vi "cm2nm_index_fiducials.vi"(2 "CurrentSessionCollectionOfPoints":T1[](array[typedef]), 4 "ReferenceSessionCollectionOfPoints":T1[](array[typedef]), 5 "IndexCurrentSession_PairingList":i32[](array[numeric]), 6 "ReplacePairedFidName":bool, 9 "IndexRefrenceSession_PairlingList":i32[](array[numeric])) -> (0 "CurrentSessionOut":T1[](array[typedef])=[{"MetaDataFile"=path "", "X"=-1.1, "Y"=0.0, "Z"=0.0, "Group"=0, "Rotation"=0.0, "Fiducial"=TRUE, "Magnification"=0.0, "Working_Distance"=0.0, "Notes"="", "Location Name/ID"="", "OtherRelatedDataFiles"=[], "Available"=FALSE}, {"MetaDataFile"=path "", "X"=0.0, "Y"=-1.0, "Z"=0.0, "Group"=0, "Rotation"=0.0, "Fiducial"=TRUE, "Magnification"=0.0, "Working_Distance"=0.0, "Notes"="", "Location Name/ID"="", "OtherRelatedDataFiles"=[], "Available"=FALSE}, {"MetaDataFile"=path "", "X"=0.0, "Y"=1.0, "Z"=0.0, "Group"=0, "Rotation"=0.0, "Fiducial"=TRUE, "Magnification"=0.0, "Working_Distance"=0.0, "Notes"="", "Location Name/ID"="", "OtherRelatedDataFiles"=[], "Available"=FALSE}, {"MetaDataFile"=path "", "X"=1.0, "Y"=0.0, "Z"=0.0, "Group"=0, "Rotation"=0.0, "Fiducial"=TRUE, "Magnification"=0.0, "Working_Distance"=0.0, "Notes"="", "Location Name/ID"="", "OtherRelatedDataFiles"=[], "Available"=FALSE}], 1 "PairedFiducialNames":T2(array[cluster]), 3 "PairedFiducials":T3(array[cluster]))   [LabVIEW 2011]
doc: "This Vi extracts the paired coordinates and names and puts into the format that the coordinate transform functions where created. Just book keeping."
uses:
  cm2nm_coordinate_information_v2.ctl
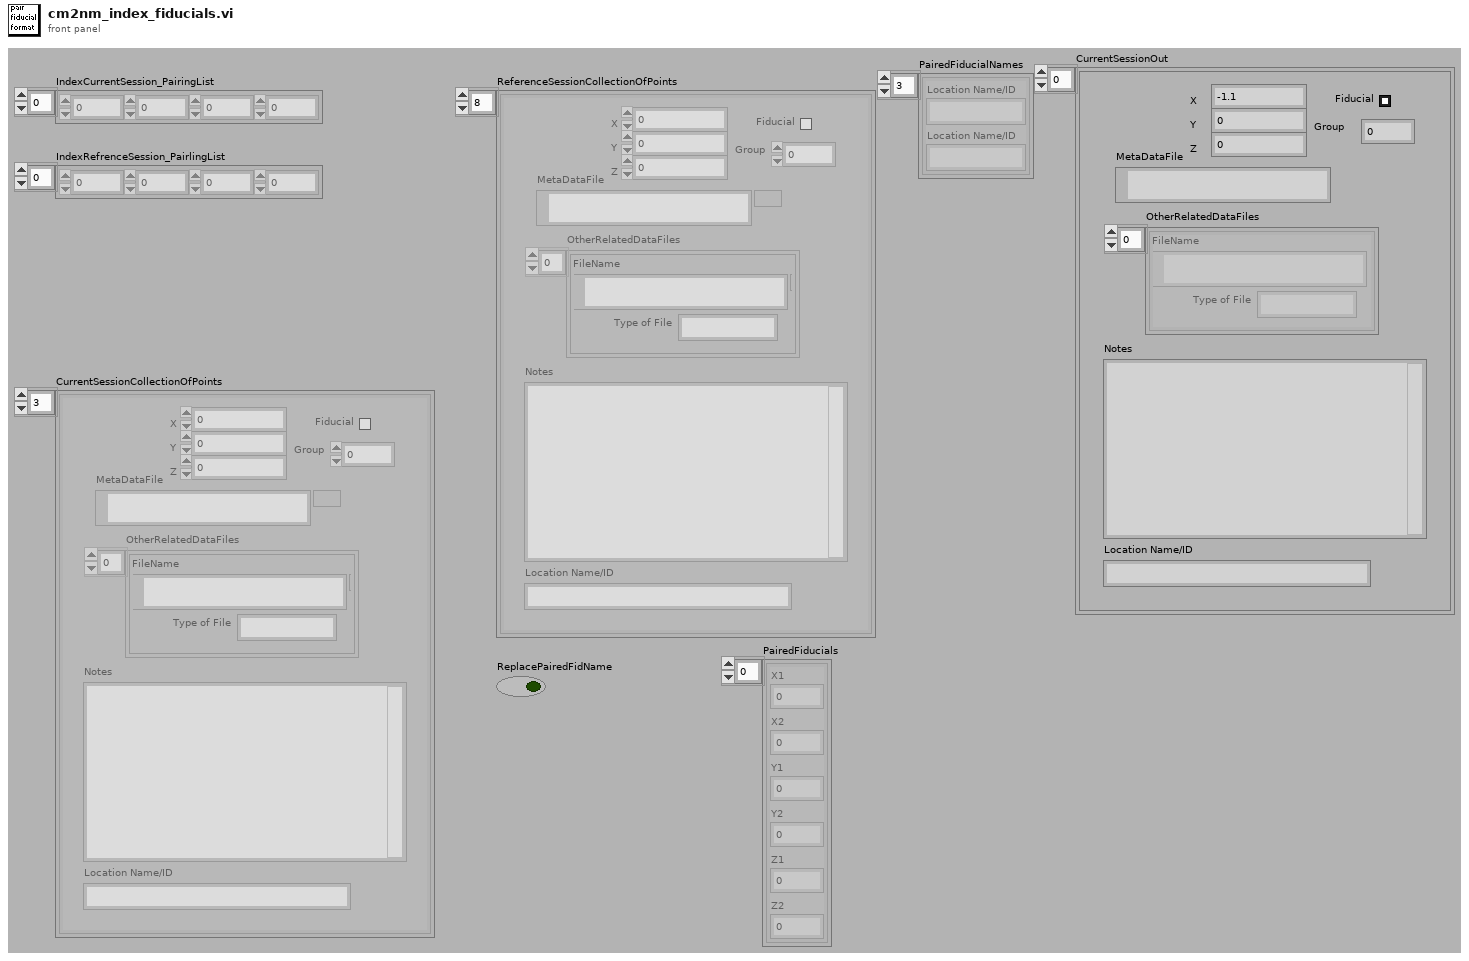
[diagram p1: front panel]
types:
  T1 = typedef "cm2nm_coordinate_information_v2.ctl" = cluster{"MetaDataFile":path, "X":dbl, "Y":dbl, "Z":dbl, "Group":i32, "Rotation":dbl[unit], "Fiducial":bool, "Magnification":dbl, "Working_Distance":dbl, "Notes":string, "Location Name/ID":string, "OtherRelatedDataFiles":cluster{"Type of File":string, "FileName":path}[], "Available":bool}
  T2 = cluster{"Location Name/ID":string, "Location Name/ID":string}[]
  T3 = cluster{"X1":dbl, "X2":dbl, "Y1":dbl, "Y2":dbl, "Z1":dbl, "Z2":dbl}[]
  T4 = cluster{"X1":dbl, "X2":dbl, "Y1":dbl, "Y2":dbl, "Z1":dbl, "Z2":dbl}
  T5 = cluster{"Location Name/ID":string, "Location Name/ID":string}
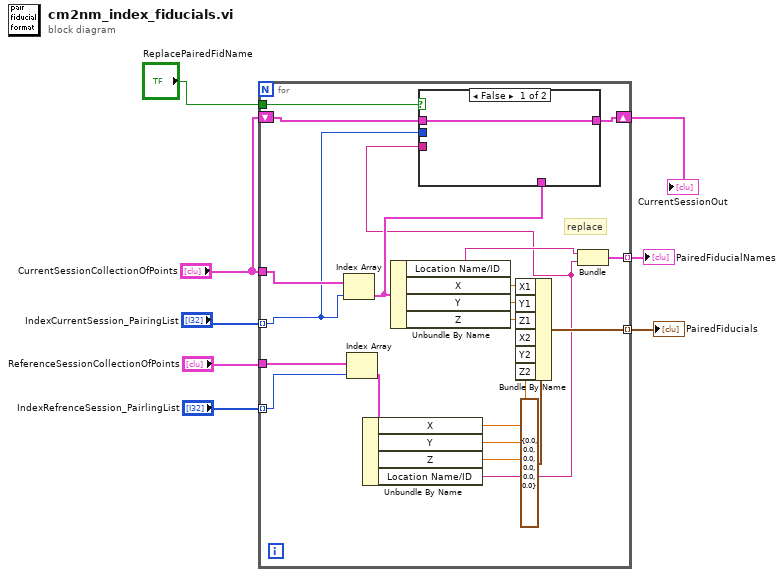
[diagram p0: block diagram]
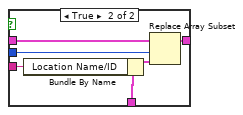
[diagram p2: hidden frame]
diagram:
  n1 = for {
    tunnel: "IndexRefrenceSession_PairlingList" -> [w9] mode=indexing
    tunnel: "IndexCurrentSession_PairingList" -> [w10] mode=indexing
    tunnel: "CurrentSessionCollectionOfPoints" -> [w16]
    tunnel: "ReferenceSessionCollectionOfPoints" -> [w28]
    tunnel: [w19] -> w8 mode=indexing
    tunnel: [w17] -> w4 mode=indexing
    shift-right: [w12] -> w2
    shift-left: "CurrentSessionCollectionOfPoints" -> [w15]
    tunnel: "ReplacePairedFidName" -> [w11]
    # "replace"
    n2 = Index Array(array=w16, index=w10) -> (element=w14:T1)
    n3 = Index Array(array=w28, index=w9) -> (element=w27:T1)
    n4 = Unbundle By Name(w27) -> ("X"=w23:dbl, "Y"=w22:dbl, "Z"=w21:dbl, "Location Name/ID"=w13:string)
    n5 = Unbundle By Name(w14) -> ("Location Name/ID"=w18:string, "X"=w26:dbl, "Y"=w25:dbl, "Z"=w24:dbl)
    n6 = case shown="False" w11 {
      tunnel: w10 -> [_ w35]
      tunnel: w15 -> [w29 w34]
      tunnel: w14 -> [_ w33]
      tunnel: w13 -> [_ w31]
      tunnel: [w29 w30] -> w12
      frame False {
      }
      frame True {
        n7 = Bundle By Name(cluster=w33, "Location Name/ID"=w31) -> (w32:T1)
        n8 = Replace Array Subset(array=w34, new element=w32, index=w35) -> (w30:T1[])
      }
    }
    n9 = Bundle By Name(cluster=T4 {"X1"=0.0, "X2"=0.0, "Y1"=0.0, "Y2"=0.0, "Z1"=0.0, "Z2"=0.0} ("Cluster"), "X1"=w26, "Y1"=w25, "Z1"=w24, "X2"=w23, "Y2"=w22, "Z2"=w21) -> (w19:T4)
    n10 = Bundle("Location Name/ID"=w18, "Location Name/ID"=w13) -> (w17:T5)  [unwired: 1 out]
  }
  "PairedFiducials" <- w8
  "PairedFiducialNames" <- w4
  "CurrentSessionOut" <- w2
